vi "CreateTemperaturesDAQTask.vi"(8 "Error In":errorcluster) -> (0 "Error Out":errorcluster, 3 "Temperatures Task":refnum<k21>)   [LabVIEW 2012]
uses:
  <vilib>/DAQmx/create/channels.llb/DAQmx Create Channel (AI-Temperature-Thermocouple).vi
  <vilib>/DAQmx/configure/timing.llb/DAQmx Timing (Sample Clock).vi
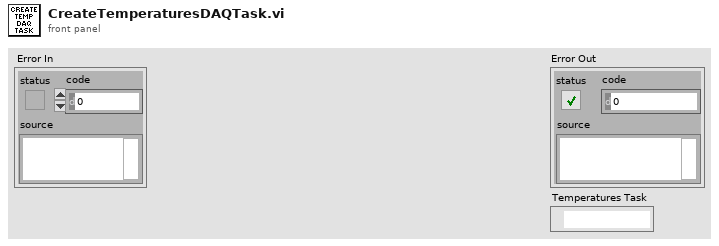
[diagram p1: front panel]
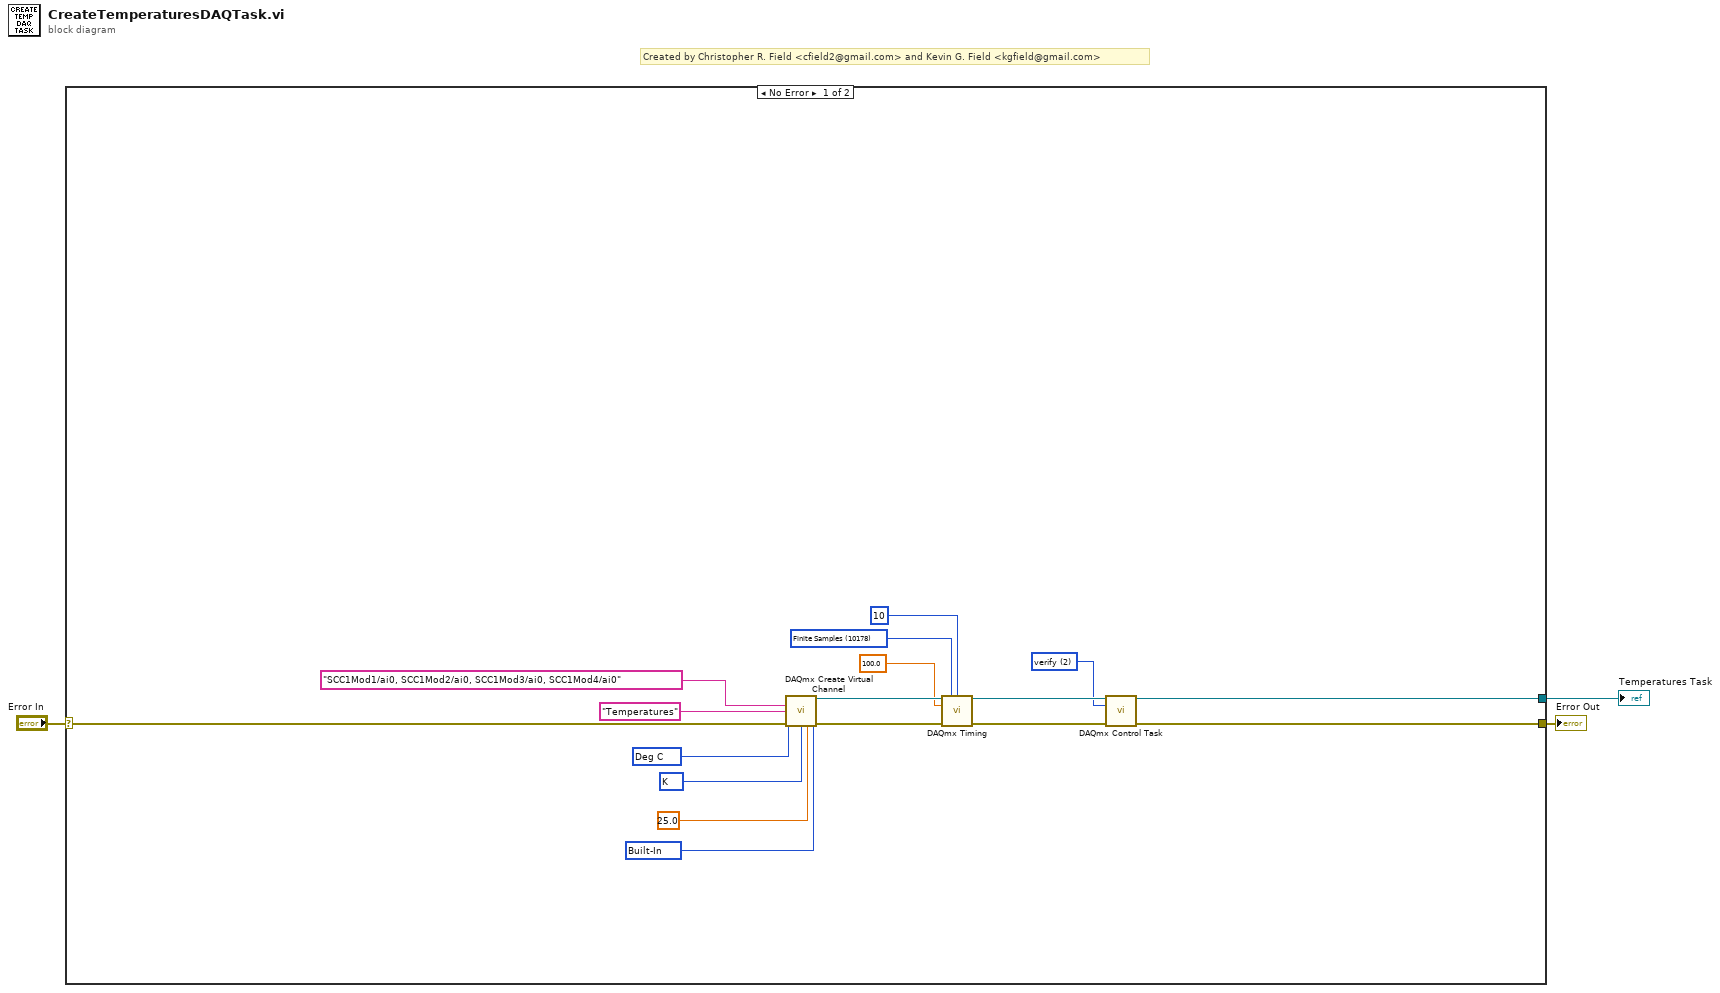
[diagram p0: block diagram]
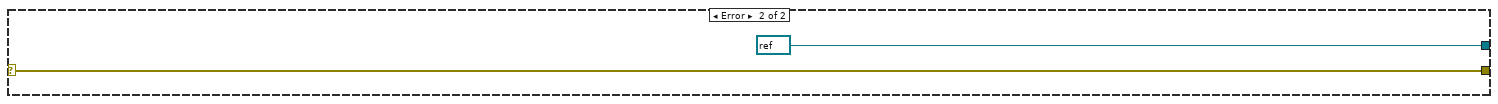
[diagram p2: hidden frame]
diagram:
  # "Created by Christopher R. Field <cfield2@gmail.com> and Kevin G. Field <kgfield@gmail.com>"
  n1 = case shown="No Error" "Error In" {
    selector: "Error In" -> [w20 w22]
    tunnel: [w19 w22] -> w2
    tunnel: [w18 refnum<k21> refnum ("task out")] -> w1
    frame No Error {
      w5 = 2 items=["verify"=2, "reserve"=4, "commit"=3, "unreserve"=5, "abort"=6] ("action")
      w9 = 10178 items=["Finite Samples"=10178, "Continuous Samples"=10123, "Hardware Timed Single Point"=12522] ("sample mode")
      w11 = 10200 items=["Built-In"=10200, "Constant Value"=10116, "Channel"=10113] ("cjc source")
      w14 = 10143 items=["Deg C"=10143, "Deg F"=10144, "Kelvins"=10325, "Deg R"=10145, "From Custom Scale"=10065] ("units")
      w15 = 10073 items=["J"=10072, "K"=10073, "N"=10077, "R"=10082, "S"=10085, "T"=10086, "B"=10047, "E"=10055] ("thermocouple type")
      n2 = call-poly <vilib>:"DAQmx Create Virtual Channel.vi"("physical channels"=tag "SCC1Mod1/ai0, SCC1Mod2/ai0, SCC1Mod3/ai0, SCC1Mod4/ai0", "cjc source"=w11, "name to assign"="Temperatures", "units"=w14, "error in"=w20, "thermocouple type"=w15, "cjc value"=25.0) -> ("task out"=w17:refnum<k21>, "error out"=w16:errorcluster)  [unwired: 7 in]
      n3 = call-poly <vilib>:"DAQmx Timing.vi"("task/channels in"=w17, "sample mode"=w9, "samples per channel"=10, "rate"=100.0, "error in"=w16) -> ("task out"=w7:refnum<k21>, "error out"=w6:errorcluster)  [unwired: 9 in]
      n4 = call <vilib>:"DAQmx Control Task.vi"("task/channels in"=w7, "action"=w5, "error in"=w6) -> ("task out"=w18:refnum<k21>, "error out"=w19:errorcluster)  [unwired: 11 in]
    }
    frame Error {
    }
  }
  "Error Out" <- w2
  "Temperatures Task" <- w1
